vi "Create html index.vi"(6 "Design exists":bool, 8 "error in":errorcluster, 9 "progress":cluster{"Progress":u8, "AC variable":string} {"Progress" scale=0.0..100.0}, 10 "Under construction":bool, 11 "DesignRequest":T1) -> (0 "error out":errorcluster, 3 "DesignRequest out":T1)   [LabVIEW 2012, in "Design Server.lvlib"]
uses:
  Design Server.lvlib
  Design Request.ctl
  Variable cluster.ctl
  RequestKeys.ctl
panel:
  out "Publish files":string[](array[string])
  out "filenames":string[](array[string])
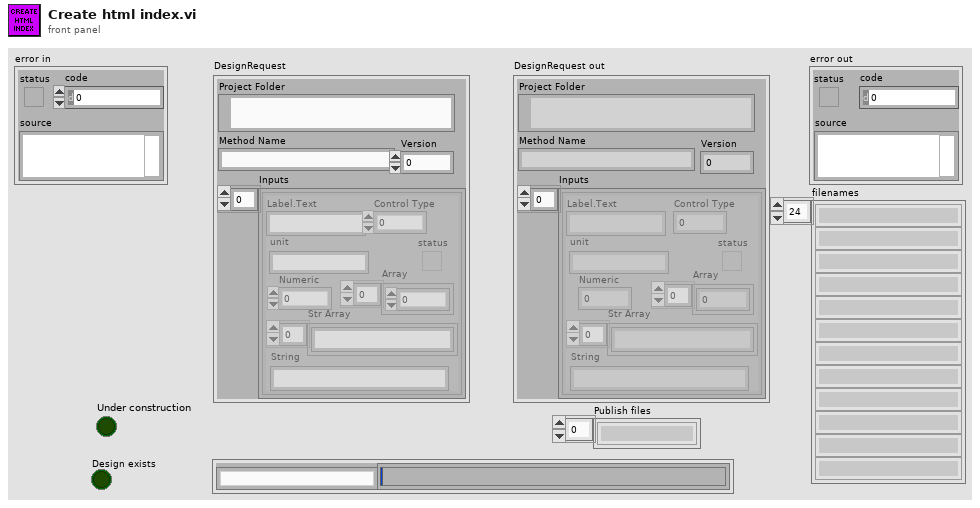
[diagram p1: front panel]
types:
  T1 = typedef "Design Server.lvlib/Design Request.ctl" = cluster{"Project Folder":path, "Method Name":string, "Inputs":T2, "Version":i32}
  T2 = typedef "Design Server.lvlib/Variable cluster.ctl" = cluster{"Label.Text":string, "Control Type":u32, "Numeric":dbl, "Array":dbl[], "status":bool, "Str Array":string[], "String":string, "unit":string}[]
  T3 = typedef "Design Server.lvlib/RequestKeys.ctl" = enum16{"FormName", "Name", "Email", "Organization", "Country", "ProjectTitle", "ProjectCity", "ProjectState", "ProjectNotes"}
  T4 = enum16{"open", "replace", "create", "open or create", "replace or create", "replace or create with confirmation"}
  T5 = typedef "Method.ctl" = cluster{"Title":string, "About":string, "Input Parameters":cluster{"Description":string, "Name":string, "Min":string, "Max":string, "Default":string, "Units":string, "Increment":string, "Stock designs":string[]}[], "AutoCAD drawings":cluster{"File Name":string, "AC Variables":string[]}[], "Stock file names":string[], "Publish files":string[], "Display images":string[]}
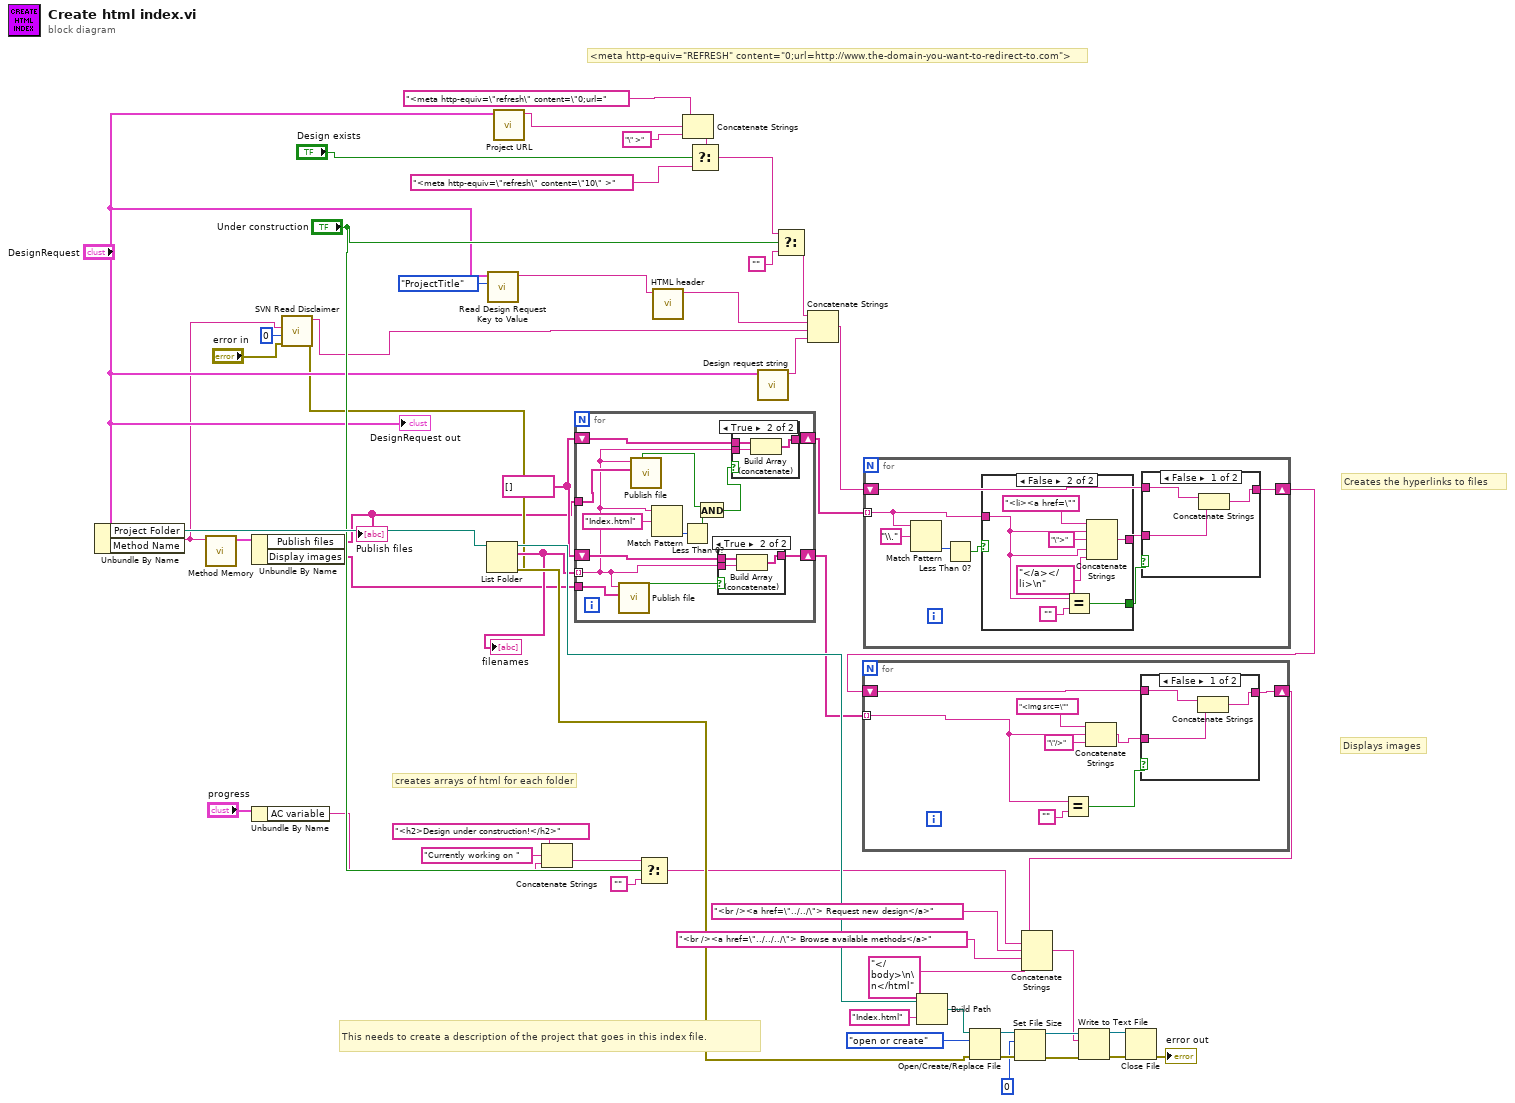
[diagram p0: block diagram]
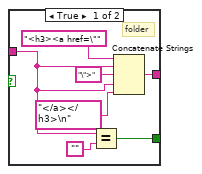
[diagram p5: hidden frame]
diagram:
  w37 = string[] []
  # "<meta http-equiv=\"REFRESH\" content=\"0;url=http://www.the-domain-you-want-to-redirect-to.com\">"
  # "Displays images"
  # "Creates the hyperlinks to files"
  # "This needs to create a description of the project that goes in this index file."
  # "creates arrays of html for each folder"
  n1 = Unbundle By Name("DesignRequest") -> ("Project Folder"=w44:path, "Method Name"=w3:string)
  n2 = call "Method Memory.vi"("Method Name"=w3) -> ("Method Out"=w4:T5)  [unwired: 8 in, 2 out]
  n3 = Unbundle By Name(w4) -> ("Publish files"=w1:string[], "Display images"=w2:string[])
  "Publish files" <- w1
  n4 = Unbundle By Name("progress") -> ("AC variable"=w22:string)
  n5 = call "SVN Read Disclaimer.vi"("error in (no error)"="error in", "Method version"=0, "Method Name"=w3) -> ("error out"=w5:errorcluster, "Disclaimer text"=w7:string)  [unwired: 6 in, 1 out]
  n6 = List Folder(path=w44, error in=w5) -> (path out=w43:path, filenames=w39:string[], error out=w42:errorcluster)  [unwired: 2 in, 1 out]
  "filenames" <- w39
  n7 = call "Read Design Request Key to Value.vi"("Request Keys"=RequestKeys."ProjectTitle", "DesignRequest"="DesignRequest") -> ("Value"=w21:string)  [unwired: 9 in]
  n8 = call "Project URL.vi"("DesignRequest"="DesignRequest") -> ("Project URL"=w13:string)  [unwired: 9 in, 1 out]
  n9 = Concatenate Strings("<h2>Design under construction!</h2>" ("t"), "Currently working on " ("string"), w22) -> (w25:string)
  n10 = for {
    shift-right: [w68] -> w35
    shift-left: w37 -> [w67]
    tunnel: w39 -> [w58] mode=indexing
    shift-right: [w66] -> w36
    shift-left: w37 -> [w65]
    tunnel: w1 -> [w60]
    tunnel: w2 -> [w56]
    n11 = call "Publish file.vi"("Publish files"=w56, "filename"=w58) -> ("Yes"=w57:bool)  [unwired: 9 in]
    n12 = call "Publish file.vi"("Publish files"=w60, "filename"=w58) -> ("Yes"=w59:bool)  [unwired: 9 in]
    n13 = Match Pattern(string=w58, regular expression="Index.html") -> (offset past match=w63:i32)  [unwired: 1 in, 3 out]
    n14 = Less Than 0?(x=w63) -> (x < 0?=w62:bool)
    n15 = And(x=w59, y=w62) -> (x .and. y?=w61:bool)
    n16 = case shown="True" w57 {
      tunnel: w58 -> [_ w76]
      tunnel: [w73 w75] -> w68
      tunnel: w67 -> [w73 w74]
      frame False {
      }
      frame True {
        n17 = Build Array (concatenate)(w74, w76) -> (w75:string[])
      }
    }
    n18 = case shown="True" w61 {
      tunnel: w58 -> [_ w72]
      tunnel: [w69 w71] -> w66
      tunnel: w65 -> [w69 w70]
      frame False {
      }
      frame True {
        n19 = Build Array (concatenate)(w70, w72) -> (w71:string[])
      }
    }
  }
  n20 = Select(t=w25, s="Under construction", f="") -> (s? t:f=w26:string)
  n21 = call "HTML header.vi"("Title"=w21) -> ("HTML header"=w20:string)  [unwired: 10 in]
  n22 = Concatenate Strings("<meta http-equiv=\"refresh\" content=\"0;url=", w13, "\" >") -> (w15:string)
  n23 = Select(t=w15, s="Design exists", f="<meta http-equiv=\"refresh\" content=\"10\" >") -> (s? t:f=w17:string)
  n24 = call "Design request string.vi"("DesignRequest"="DesignRequest") -> ("String"=w38:string)  [unwired: 9 in, 1 out]
  n25 = Select(t=w17, s="Under construction", f="") -> (s? t:f=w31:string)
  n26 = Concatenate Strings(w31, w20, w7, w38) -> (w45:string)
  n27 = for {
    tunnel: w36 -> [w80] mode=indexing
    shift-right: [w84] -> w34
    shift-left: w45 -> [w82]
    n28 = Match Pattern(string=w80, regular expression="\\.") -> (offset past match=w79:i32)  [unwired: 1 in, 3 out]
    n29 = Less Than 0?(x=w79) -> (x < 0?=w78:bool)
    n30 = case shown="False" w78 {
      tunnel: [w89 w96] -> w83
      tunnel: w80 -> [w86 w93]
      tunnel: [w85 w92] -> w81
      frame True {
        # "folder"
        n31 = Equal?(x=w86, y="") -> (x = y?=w85:bool)
        n32 = Concatenate Strings("<h3><a href=\"" ("string"), w86, "\">" ("string"), w86, "</a></h3>\n" ("string")) -> (w89:string)
      }
      frame False {
        n33 = Equal?(x=w93, y="") -> (x = y?=w92:bool)
        n34 = Concatenate Strings("<li><a href=\"" ("string"), w93, "\">" ("string"), w93, "</a></li>\n" ("string")) -> (w96:string)
      }
    }
    n35 = case shown="False" w81 {
      tunnel: [w101 w102] -> w84
      tunnel: w83 -> [w100 _]
      tunnel: w82 -> [w99 w102]
      frame False {
        n36 = Concatenate Strings(w99, w100) -> (w101:string)
      }
      frame True {
      }
    }
  }
  n37 = for {
    tunnel: w35 -> [w106] mode=indexing
    shift-right: [w110] -> w33
    shift-left: w34 -> [w108]
    n38 = Equal?(x=w106, y="") -> (x = y?=w107:bool)
    n39 = Concatenate Strings("<img src=\"" ("string"), w106, "\"/>" ("string")) -> (w109:string)
    n40 = case shown="False" w107 {
      tunnel: [w113 w114] -> w110
      tunnel: w109 -> [w112 _]
      tunnel: w108 -> [w111 w114]
      frame False {
        n41 = Concatenate Strings(w111, w112) -> (w113:string)
      }
      frame True {
      }
    }
  }
  n42 = Build Path(base path=w43, name or relative path="Index.html") -> (appended path=w54:path)
  n43 = Open/Create/Replace File(file path (use dialog)=w54, error in=w42, operation (0:open)=T4."open or create") -> (refnum out=w50:refnum<file>, error out=w48:errorcluster)  [unwired: 3 in, 1 out]
  n44 = Set File Size(4:w48, 6:i64 0 ("size (in bytes)"), 7:w50) -> (0:w47:errorcluster, 3:w49:refnum<file>)
  n45 = Concatenate Strings(w33, w26, "<br /><a href=\"../../\"> Request new design</a>" ("string"), "<br /><a href=\"../../../\"> Browse available methods</a>" ("string"), "</body>\n\n</html") -> (w30:string)
  n46 = Write to Text File(file (use dialog)=w49, text=w30, error in=w47) -> (refnum out=w51:refnum<file>, error out=w52:errorcluster)  [unwired: 1 in, 1 out]
  n47 = Close File(refnum=w51, error in=w52) -> (error out=→"error out":errorcluster)  [unwired: 1 out]
  "DesignRequest out" <- "DesignRequest"
